vi "2039 PID_GoDistance.vi"() -> ()   [LabVIEW 2016, in "2039lib.lvlib"]
uses:
  2039lib.lvlib
  <vilib>/Rock Robotics/WPI/MotorControl/WPI_MotorControlDeviceRef.ctl
  <vilib>/Rock Robotics/WPI/MotorControl/WPI_MotorControlType.ctl
  <vilib>/Rock Robotics/SystemInterfaces/DIO/FPGA_DIOPWMChannel.ctl
  <vilib>/Rock Robotics/WPI/PWM/WPI_PWMDeadband.ctl
  <vilib>/addons/control/pid/pid.llb/PID (DBL).vi
  <vilib>/addons/control/pid/NI_PID_pid.lvlib
panel:
  out "output":dbl format="%.2f"
  in  "PID gains":T1={"proportional gain (Kc)"=1.0, "integral time (Ti, min)"=0.01, "derivative time (Td, min)"=0.0} {"derivative time (Td, min)" format="%.3f"; "integral time (Ti, min)" format="%.3f"; "proportional gain (Kc)" format="%.3f"}
  in  "CAN Talon SRX Ref Array":T2[](array[typedef])
  in  "Desired Distance (ft)":dbl
  in  "Wheel Radius (in)":dbl
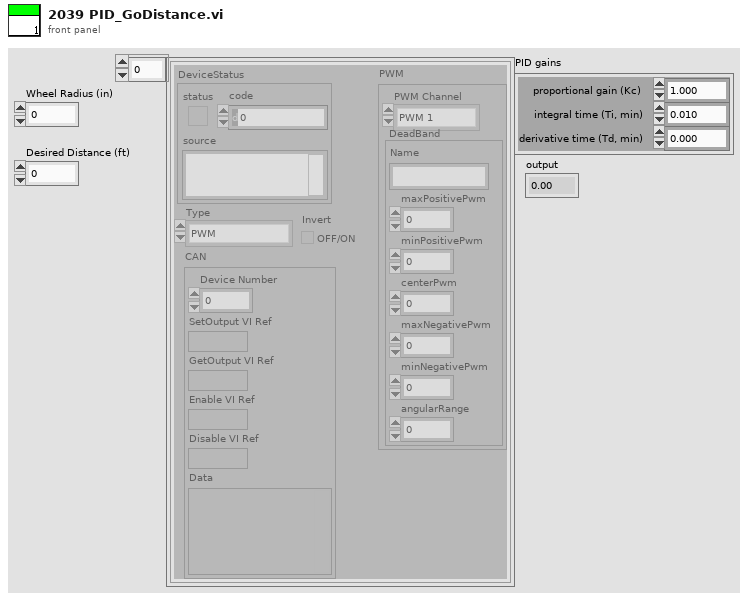
[diagram p1: front panel]
types:
  T1 = cluster{"proportional gain (Kc)":dbl, "integral time (Ti, min)":dbl, "derivative time (Td, min)":dbl}
  T2 = typedef "WPI_MotorControlDeviceRef.ctl" = cluster{"DeviceStatus":errorcluster, "Type":T3, "PWM":cluster{"PWM Channel":T4, "DeadBand":T5}, "CAN":cluster{"Device Number":u8, "SetOutput VI Ref":variant, "GetOutput VI Ref":variant, "Enable VI Ref":variant, "Disable VI Ref":variant, "Data":variant}, "Invert":bool}
  T3 = typedef "WPI_MotorControlType.ctl" = enum16{"PWM", "CAN"}
  T4 = typedef "FPGA_DIOPWMChannel.ctl" = enum8{"PWM 0", "PWM 1", "PWM 2", "PWM 3", "PWM 4", "PWM 5", "PWM 6", "PWM 7", "PWM 8", "PWM 9", "PWM MXP 0", "PWM MXP 1", "PWM MXP 2", "PWM MXP 3", "PWM MXP 4", "PWM MXP 5", "PWM MXP 6", "PWM MXP 7", "PWM MXP 8", "PWM MXP 9", "Invalid"}
  T5 = typedef "WPI_PWMDeadband.ctl" = cluster{"Name":string, "maxPositivePwm":i32, "minPositivePwm":i32, "centerPwm":i32, "maxNegativePwm":i32, "minNegativePwm":i32, "angularRange":u16}
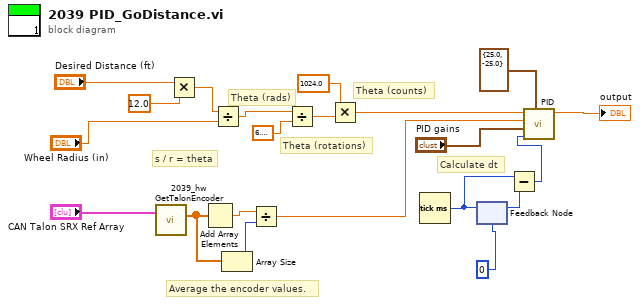
[diagram p0: block diagram]
diagram:
  # "Average the encoder values."
  # "Calculate dt"
  # "Theta (counts)"
  # "Theta (rotations)"
  # "Theta (rads)"
  # "s / r = theta"
  n1 = call "2039_hw GetTalonEncoder.vi"("CAN Talon SRX Ref Array"="CAN Talon SRX Ref Array") -> ("Encoder Position Array"=w6:dbl[])  [unwired: 1 in, 3 out]
  n2 = Multiply(x="Desired Distance (ft)", y=12.0) -> (x*y=w18:dbl)
  n3 = Add Array Elements(numeric array=w6) -> (sum=w7:dbl)
  n4 = Divide(x=w18, y="Wheel Radius (in)") -> (x/y=w16:dbl)
  n5 = Array Size(array=w6) -> (size(s)=w5:i32)
  n6 = Divide(x=w7, y=w5) -> (x/y=w4:dbl)
  n7 = Divide(x=w16, y=6.283185307179586) -> (x/y=w14:dbl)
  n8 = Multiply(x=1024.0, y=w14) -> (x*y=w12:dbl)
  n9 = Tick Count (ms)() -> (millisecond timer value=w9:u32)
  n10 = feedback-in #1(w9) -> ()
  n11 = feedback #1(0) -> (w10:u32)
  n12 = Subtract(x=w9, y=w10) -> (x-y=w8:u32)
  n13 = call-poly <vilib>:"PID.vi"("output range"=cluster{"output high":dbl, "output low":dbl} {"output high"=25.0, "output low"=-25.0}, "dt (s)"=w8, "PID gains"="PID gains", "process variable"=w4, "setpoint"=w12) -> ("output"=→"output":dbl)  [unwired: 5 in, 1 out]
